vi "HD_Config.vi"(8 "error in (no error)":errorcluster, 10 "HD Config in":T1, 11 "Step":enum16{"Initial", "Write", "Read"}(ring)) -> (0 "error out":errorcluster, 3 "HD Config out":T1)   [LabVIEW 2017]
uses:
  Ctrls/HD Config.ctl
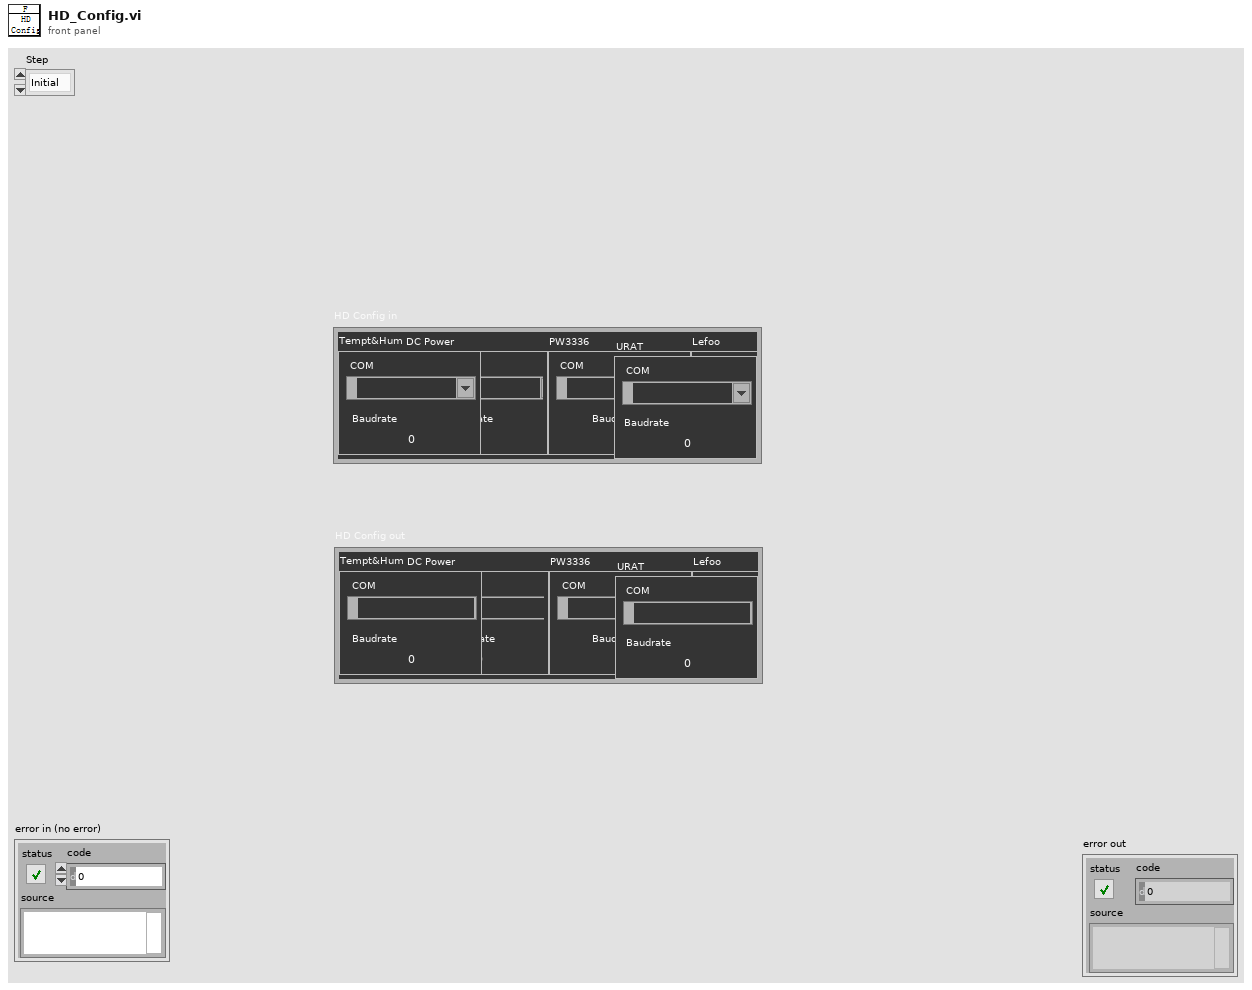
[diagram p1: front panel]
types:
  T1 = typedef "HD Config.ctl" = cluster{" PC":cluster{"PC Address":u8[], "PC Port":i32}, "FCO":cluster{"COM":refnum<visa-resource-name>, "Baudrate":u32}, "DC Power ":cluster{"COM":refnum<visa-resource-name>, "Baudrate":u32}, "PW3336":cluster{"COM":refnum<visa-resource-name>, "Baudrate":u32}, "Lefoo":cluster{"COM":refnum<visa-resource-name>, "Baudrate":u32}, "Tempt&Hum":cluster{"COM":refnum<visa-resource-name>, "Baudrate":u32}, "DIPC":cluster{"COM":refnum<visa-resource-name>}, "Daemon":cluster{"IP Address":string, "Port":u16, "Retry":u16}, "URAT":cluster{"COM":refnum<visa-resource-name>, "Baudrate":u32}, "Fail_resume_mode":bool, "GRR":bool}
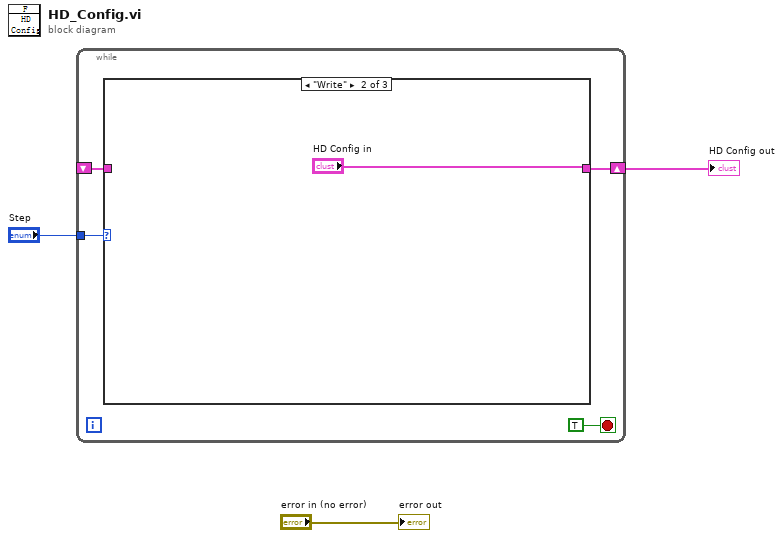
[diagram p0: block diagram]
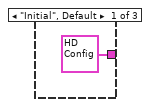
[diagram p2: hidden frame]
diagram:
  n1 = while {
    tunnel: "Step" -> [w6]
    shift-right: [w5] -> w1
    shift-left: _ -> [w4]
    stop <- TRUE stop-if-true
    n2 = case shown="\"Write\"" w6 {
      tunnel: [T1 {" PC"={"PC Address"=[], "PC Port"=0}, "FCO"={"COM"="", "Baudrate"=0}, "DC Power "={"COM"="", "Baudrate"=0}, "PW3336"={"COM"="", "Baudrate"=0}, "Lefoo"={"COM"="", "Baudrate"=0}, "Tempt&Hum"={"COM"="", "Baudrate"=0}, "DIPC"={"COM"=""}, "Daemon"={"IP Address"="", "Port"=0, "Retry"=0}, "URAT"={"COM"="", "Baudrate"=0}, "Fail_resume_mode"=FALSE, "GRR"=FALSE} ("HD Config in") "HD Config in" w10] -> w5
      tunnel: w4 -> [_ _ w10]
      frame "Initial", Default {
      }
      frame "Write" {
      }
      frame "Read" {
      }
    }
  }
  "HD Config out" <- w1
  "error out" <- "error in (no error)"
